vi "Get RIOs for APU.vi"(8 "error in (no error)":errorcluster, 10 "APU name":string, 11 "Item Ref in":T1 format="%.0x") -> (0 "error out":errorcluster, 2 "RIO Addresses":string[](array[string]), 3 "Item Ref out":T1 format="%.0x")   [LabVIEW 2020, in "Engine Simulation Toolkit System Explorer.lvlib"]
uses:
  Engine Simulation Toolkit System Explorer.lvlib
  <vilib>/NI VeriStand/Custom Device API/Custom Device Item Ref.ctl
  Shared/Properties.vi
  <vilib>/NI VeriStand/Custom Device API/Get Item Property (String Array).vi
  <vilib>/NI VeriStand/Custom Device API/Custom Device API.lvlib
  Shared/Engine Simulation Toolkit Shared.lvlib
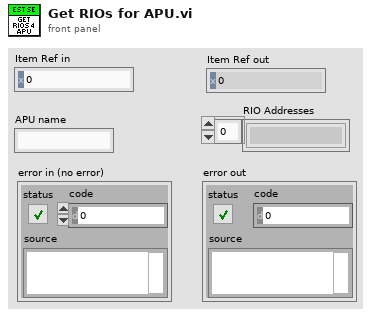
[diagram p1: front panel]
types:
  T1 = typedef "Custom Device API.lvlib/Custom Device Item Ref.ctl" = u64
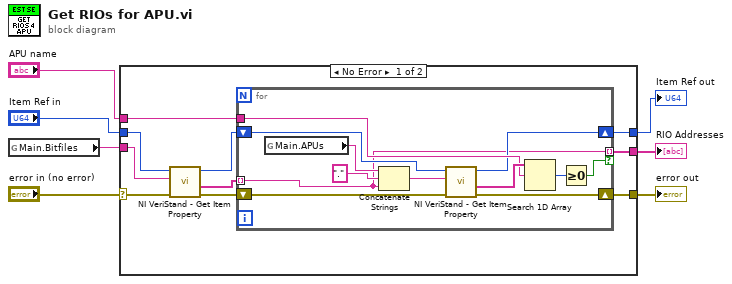
[diagram p0: block diagram]
diagram:
  n1 = global read "Properties.vi" "Main.Bitfiles"() -> (w7:string)
  n2 = case shown="No Error" "error in (no error)" {
    selector: "error in (no error)" -> [w12 w31]
    tunnel: w7 -> [w17 _]
    tunnel: "Item Ref in" -> [w14 w30]
    tunnel: [w11 w31] -> w4
    tunnel: [w10 _] -> w3
    tunnel: "APU name" -> [w9 _]
    tunnel: [w8 w30] -> w1
    frame No Error {
      n3 = call-poly <vilib>:"NI VeriStand - Get Item Property.vi"("error in (no error)"=w12, "Property Name"=w17, "Item Ref in"=w14) -> ("error out"=w13:errorcluster, "Value"=w16:string[], "Item Ref out"=w15:T1)  [unwired: 5 in, 1 out]
      n4 = for {
        tunnel: w9 -> [w27]
        tunnel: [w19] -> w10 mode=indexing if=w26
        shift-right: [w24] -> w11
        shift-left: w13 -> [w25]
        tunnel: w16 -> [w19] mode=indexing
        shift-right: [w22] -> w8
        shift-left: w15 -> [w23]
        n5 = global read "Properties.vi" "Main.APUs"() -> (w20:string)
        n6 = Concatenate Strings(w20, "." ("string"), w19) -> (w18:string)
        n7 = call-poly <vilib>:"NI VeriStand - Get Item Property.vi"("error in (no error)"=w25, "Property Name"=w18, "Item Ref in"=w23) -> ("error out"=w24:errorcluster, "Value"=w29:string[], "Item Ref out"=w22:T1)  [unwired: 5 in, 1 out]
        n8 = Search 1D Array(1D array=w29, element=w27) -> (index of element=w28:i32)  [unwired: 1 in]
        n9 = Greater Or Equal To 0?(x=w28) -> (x >= 0?=w26:bool)
      }
    }
    frame Error {
    }
  }
  "error out" <- w4
  "RIO Addresses" <- w3
  "Item Ref out" <- w1
